vi "Initialize Tab Control.vi"(5 "Page Visible":bool, 7 "Independent Label":bool, 8 "error in":errorcluster, 9 "Only clear":bool, 11 "Array":refnum<vi>[](array[refnum])) -> (0 "error out":errorcluster)   [LabVIEW 2014]
doc: "This VI set the properties of controls located on each page of the tab control."
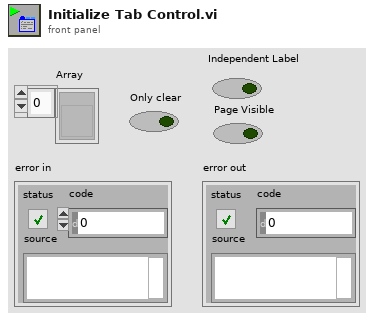
[diagram p1: front panel]
types:
  T1 = enum8{"Enabled", "Disabled", "Disabled and Grayed Out"}
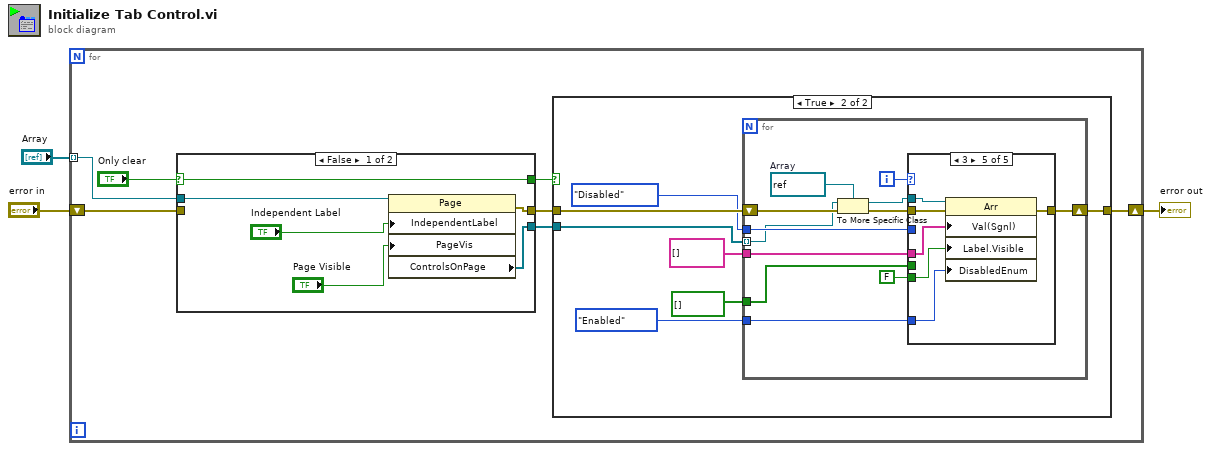
[diagram p0: block diagram]
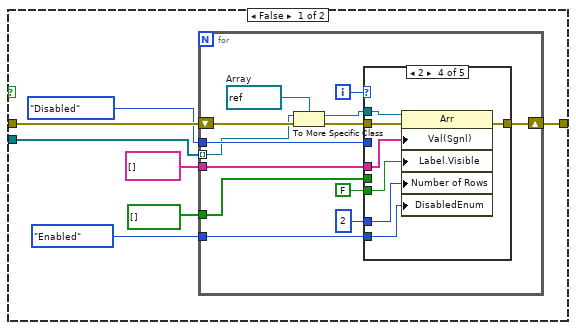
[diagram p2: hidden frame]
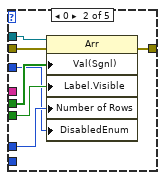
[diagram p4: hidden frame]
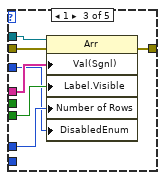
[diagram p5: hidden frame]
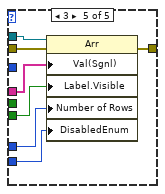
[diagram p6: hidden frame]
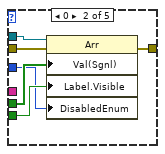
[diagram p8: hidden frame]
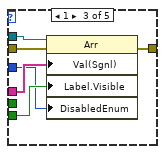
[diagram p9: hidden frame]
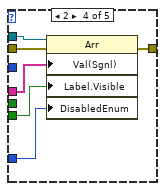
[diagram p10: hidden frame]
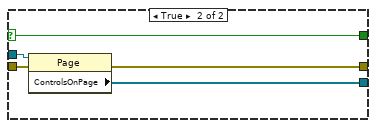
[diagram p11: hidden frame]
diagram:
  n1 = for {
    tunnel: "Array" -> [w10] mode=indexing
    shift-right: [w8] -> w2
    shift-left: "error in" -> [w5]
    n2 = case shown="False" "Only clear" {
      selector: "Only clear" -> [w104 w110]
      tunnel: w10 -> [w109 w113]
      tunnel: [w106 w112] -> w9
      tunnel: [w105 w111] -> w6
      tunnel: w5 -> [_ w114]
      tunnel: [w104 w110] -> w4
      frame False {
        n3 = property class="Page"(reference=w109, "IndependentLabel"="Independent Label", "PageVis"="Page Visible") -> (error out=w106:errorcluster, "ControlsOnPage"=w105:refnum<vi>[])  [unwired: 1 in, 1 out]
      }
      frame True {
        n4 = property class="Page"(reference=w113, error in=w114) -> (error out=w112:errorcluster, "ControlsOnPage"=w111:refnum<vi>[])  [unwired: 1 out]
      }
    }
    n5 = case shown="True" w4 {
      tunnel: w9 -> [w17 w66]
      tunnel: [w14 w63] -> w8
      tunnel: w6 -> [w11 w60]
      frame False {
        n6 = for {
          shift-right: [w26] -> w14
          shift-left: w17 -> [w30]
          tunnel: string[] [] -> [w23]
          tunnel: bool[] [] -> [w22]
          tunnel: T1."Disabled" ("Disabled") -> [w20]
          tunnel: T1."Enabled" ("Disabled") -> [w19]
          tunnel: w11 -> [w18] mode=indexing
          i -> [w28]
          w29 = refnum<vi> refnum  # Array
          n7 = To More Specific Class(target class=w29, reference=w18, error in=w30) -> (specific class reference=w25:refnum<vi>, error out=w27:errorcluster)
          n8 = case shown="2" w28 {
            tunnel: w27 -> [w31 w35 w42 w49 w56]
            tunnel: [w31 w36 w43 w50 w57] -> w26
            tunnel: w25 -> [_ w37 w44 w51 w58]
            tunnel: FALSE -> [_ w38 w45 w52 w59]
            tunnel: w23 -> [_ _ w41 w48 w55]
            tunnel: w22 -> [_ w34 _ _ _]
            tunnel: u32 2 -> [_ w33 w40 w47 w54]
            tunnel: w20 -> [_ w32 w39 _ _]
            tunnel: w19 -> [_ _ _ w46 w53]
            frame -1, Default {
            }
            frame 0 {
              n9 = property class="Arr"(reference=w37, error in=w35, "Val(Sgnl)"=w34, "Label.Visible"=w38, "Number of Rows"=w33, "DisabledEnum"=w32) -> (error out=w36:errorcluster)  [unwired: 1 out]
            }
            frame 1 {
              n10 = property class="Arr"(reference=w44, error in=w42, "Val(Sgnl)"=w41, "Label.Visible"=w45, "Number of Rows"=w40, "DisabledEnum"=w39) -> (error out=w43:errorcluster)  [unwired: 1 out]
            }
            frame 2 {
              n11 = property class="Arr"(reference=w51, error in=w49, "Val(Sgnl)"=w48, "Label.Visible"=w52, "Number of Rows"=w47, "DisabledEnum"=w46) -> (error out=w50:errorcluster)  [unwired: 1 out]
            }
            frame 3 {
              n12 = property class="Arr"(reference=w58, error in=w56, "Val(Sgnl)"=w55, "Label.Visible"=w59, "Number of Rows"=w54, "DisabledEnum"=w53) -> (error out=w57:errorcluster)  [unwired: 1 out]
            }
          }
        }
      }
      frame True {
        n13 = for {
          shift-right: [w74] -> w63
          shift-left: w66 -> [w78]
          tunnel: string[] [] -> [w71]
          tunnel: bool[] [] -> [w70]
          tunnel: T1."Disabled" ("Disabled") -> [w69]
          tunnel: T1."Enabled" ("Disabled") -> [w68]
          tunnel: w60 -> [w67] mode=indexing
          i -> [w76]
          w77 = refnum<vi> refnum  # Array
          n14 = To More Specific Class(target class=w77, reference=w67, error in=w78) -> (specific class reference=w73:refnum<vi>, error out=w75:errorcluster)
          n15 = case shown="3" w76 {
            tunnel: w75 -> [w79 w82 w88 w94 w100]
            tunnel: [w79 w83 w89 w95 w101] -> w74
            tunnel: w73 -> [_ w84 w90 w96 w102]
            tunnel: FALSE -> [_ w85 w91 w97 w103]
            tunnel: w71 -> [_ _ w87 w93 w99]
            tunnel: w70 -> [_ w81 _ _ _]
            tunnel: w69 -> [_ w80 w86 _ _]
            tunnel: w68 -> [_ _ _ w92 w98]
            frame -1, Default {
            }
            frame 0 {
              n16 = property class="Arr"(reference=w84, error in=w82, "Val(Sgnl)"=w81, "Label.Visible"=w85, "DisabledEnum"=w80) -> (error out=w83:errorcluster)  [unwired: 1 out]
            }
            frame 1 {
              n17 = property class="Arr"(reference=w90, error in=w88, "Val(Sgnl)"=w87, "Label.Visible"=w91, "DisabledEnum"=w86) -> (error out=w89:errorcluster)  [unwired: 1 out]
            }
            frame 2 {
              n18 = property class="Arr"(reference=w96, error in=w94, "Val(Sgnl)"=w93, "Label.Visible"=w97, "DisabledEnum"=w92) -> (error out=w95:errorcluster)  [unwired: 1 out]
            }
            frame 3 {
              n19 = property class="Arr"(reference=w102, error in=w100, "Val(Sgnl)"=w99, "Label.Visible"=w103, "DisabledEnum"=w98) -> (error out=w101:errorcluster)  [unwired: 1 out]
            }
          }
        }
      }
    }
  }
  "error out" <- w2
